vi "ui_connection_status.vi"(10 "Boolean":bool, 11 "String in":refnum<vi>) -> (3 "status":string)   [LabVIEW 2011]
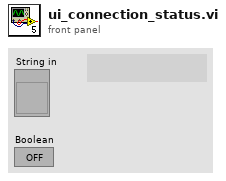
[diagram p1: front panel]
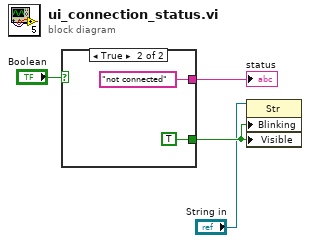
[diagram p0: block diagram]
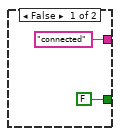
[diagram p2: hidden frame]
diagram:
  n1 = case shown="True" "Boolean" {
    tunnel: ["connected" "not connected"] -> w3
    tunnel: [FALSE TRUE] -> w4
    frame False {
    }
    frame True {
    }
  }
  "status" <- w3
  n2 = property on="Property Node" class="Str"(reference="String in", "Blinking"=w4, "Visible"=w4) -> ()  [unwired: 1 in, 2 out]
